vi "loadDotNetMember.vi"(0 "dotNetModule":refnum<k7>, 1 "Strong Assembly path":string="NationalInstruments.VeriStand.ClientAPI, Version=2.0.0.0, Culture=neutral, PublicKeyToken=a6d690c380daa308, processorArchitecture=MSIL", 2 "ClassName":string="NationalInstruments.VeriStand.ClientAPI.Factory", 3 "MemberName":string, 4 "Member token":i32, 5 "error in(no error)":errorcluster, 6 "ClassReference":string, 7 "Call Member?":i32, 9 "CreateObject":bool, 11 "Constructor Token":i32=100663484) -> (14 "dotNetModule(out)":refnum<k7>, 19 "error out":errorcluster)   [LabVIEW 2010]
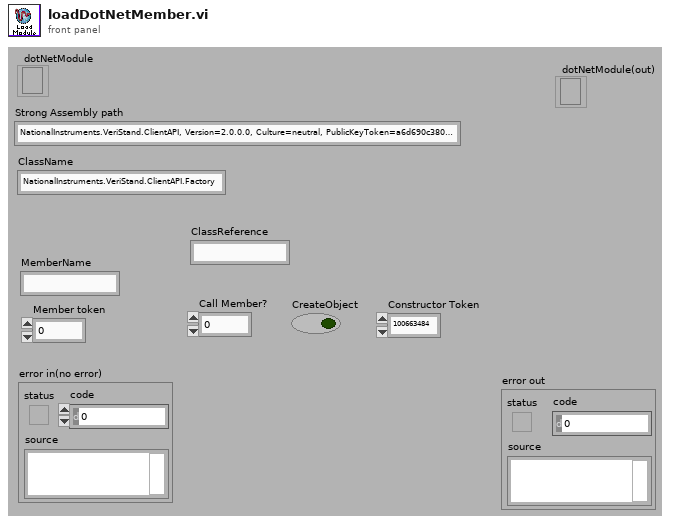
[diagram p1: front panel]
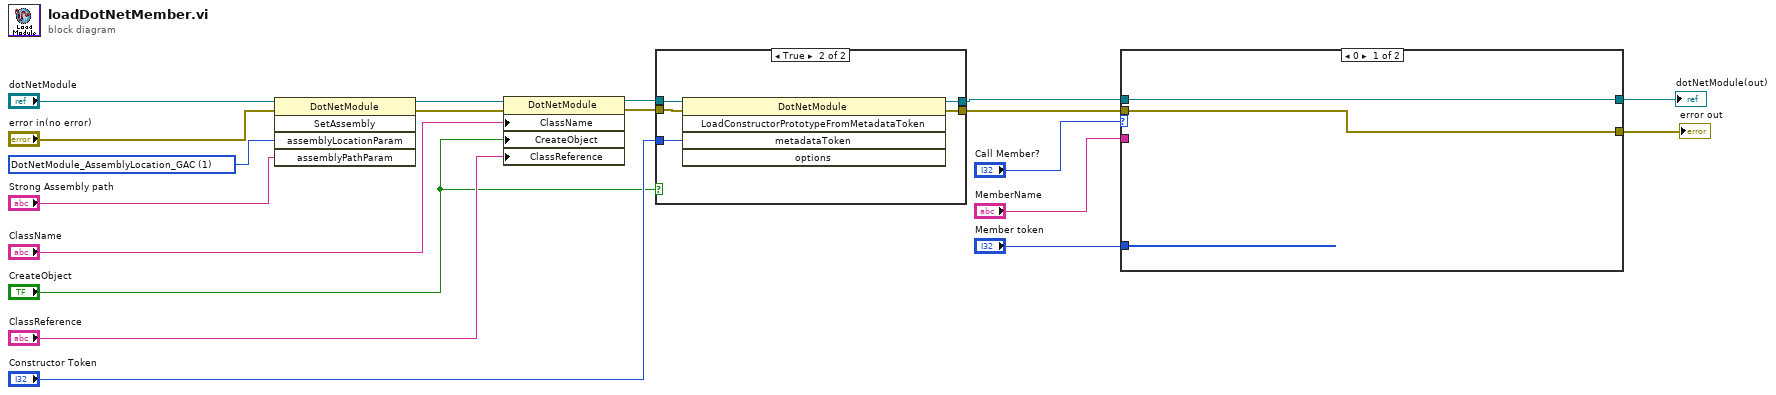
[diagram p0: block diagram]
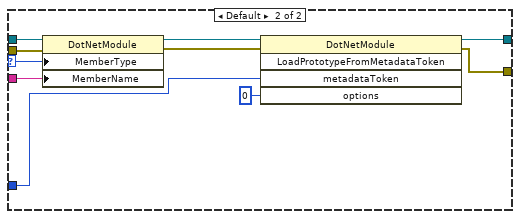
[diagram p2: hidden frame]
diagram:
  w10 = 1 items=["DotNetModule_AssemblyLocation_File", "DotNetModule_AssemblyLocation_GAC"] ("assemblyLocationParam")
  n1 = invoke class="DotNetModule" method="SetAssembly"(reference="dotNetModule", error in="error in(no error)", "assemblyLocationParam"=w10, "assemblyPathParam"="Strong Assembly path") -> (reference out=w11:refnum<k7>, error out=w12:errorcluster)  [unwired: 1 in, 3 out]
  n2 = property class="DotNetModule"(reference=w11, error in=w12, "ClassName"="ClassName", "CreateObject"="CreateObject", "ClassReference"="ClassReference") -> (reference out=w14:refnum<k7>, error out=w15:errorcluster)
  n3 = case shown="True" "CreateObject" {
    tunnel: "Constructor Token" -> [_ w26]
    tunnel: w15 -> [w20 w25]
    tunnel: w14 -> [w21 w24]
    tunnel: [w21 w23] -> w3
    tunnel: [w20 w22] -> w2
    frame False {
    }
    frame True {
      n4 = invoke class="DotNetModule" method="LoadConstructorPrototypeFromMetadataToken"(reference=w24, error in=w25, "metadataToken"=w26) -> (reference out=w23:refnum<k7>, error out=w22:errorcluster)  [unwired: 2 in, 3 out]
    }
  }
  n5 = case shown="0" "Call Member?" {
    selector: "Call Member?" -> [_ w30]
    tunnel: "Member token" -> [_ w37]
    tunnel: [w28 w36] -> w18
    tunnel: [w27 w35] -> w17
    tunnel: w3 -> [w28 w32]
    tunnel: w2 -> [w27 w31]
    tunnel: "MemberName" -> [_ w29]
    frame 0 {
    }
    frame Default {
      n6 = property class="DotNetModule"(reference=w32, error in=w31, "MemberType"=w30, "MemberName"=w29) -> (reference out=w33:refnum<k7>, error out=w34:errorcluster)
      n7 = invoke class="DotNetModule" method="LoadPrototypeFromMetadataToken"(reference=w33, error in=w34, "metadataToken"=w37, "options"=0) -> (reference out=w36:refnum<k7>, error out=w35:errorcluster)  [unwired: 1 in, 3 out]
    }
  }
  "error out" <- w17
  "dotNetModule(out)" <- w18
